vi "Configure AI Task.vi"(7 "Sampling Rate":dbl, 8 "error in (no error)":errorcluster, 11 "DAQ Tasks in":T1) -> (0 "error out":errorcluster, 3 "DAQ Tasks out":T1)   [LabVIEW 2015, in "DAQmx Module Runtime.lvclass"]
doc: "Configure AI Task by setting buffer to overwrite unread samples, setting sample clock, and starting the task."
uses:
  DAQmx Module Runtime.lvclass
  DAQ Tasks.ctl
  <vilib>/DAQmx/configure/timing.llb/DAQmx Timing (Sample Clock).vi
  <resource>/objmgr/daqmx.rc
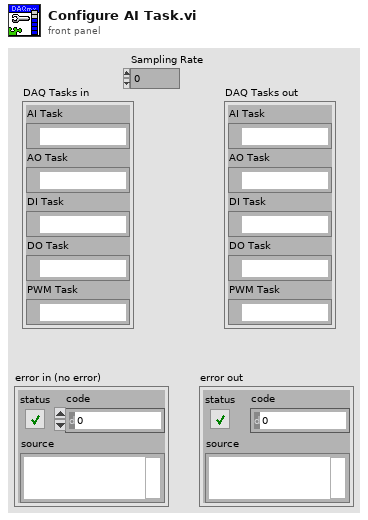
[diagram p1: front panel]
types:
  T1 = typedef "DAQmx Module Runtime.lvclass/DAQ Tasks.ctl" = cluster{"AI Task":refnum<k21>, "AO Task":refnum<k21>, "DI Task":refnum<k21>, "DO Task":refnum<k21>, "PWM Task":refnum<k21>}
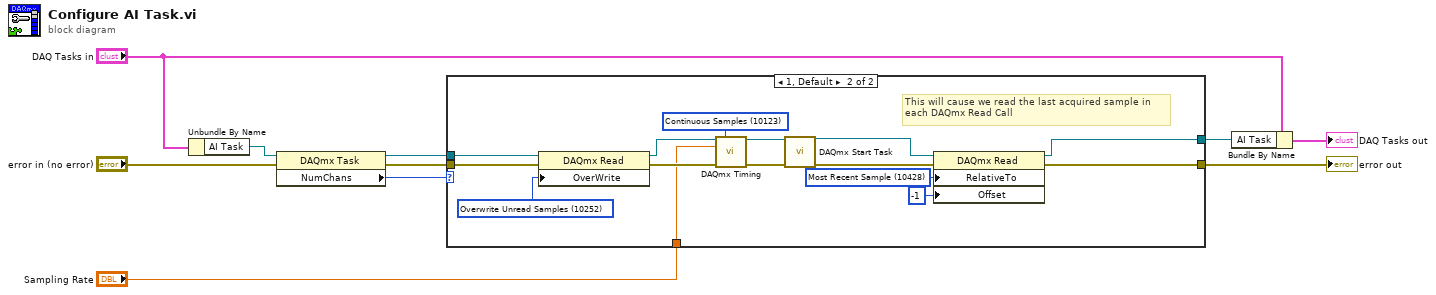
[diagram p0: block diagram]
diagram:
  n1 = Unbundle By Name("DAQ Tasks in") -> ("AI Task"=w2:refnum<k21>)
  n2 = property class="DAQmx Task"(reference=w2, error in="error in (no error)") -> (reference out=w9:refnum<k21>, error out=w7:errorcluster, "NumChans"=w6:u32)
  n3 = case shown="1, Default" w6 {
    tunnel: [w12 w14] -> w10
    tunnel: w9 -> [w11 w27]
    tunnel: w7 -> [w12 w26]
    tunnel: [w11 w13] -> w5
    tunnel: "Sampling Rate" -> [_ w19]
    frame 0 {
    }
    frame 1, Default {
      w18 = 10428 items=["First Sample"=10424, "Current Read Position"=10425, "Reference Trigger"=10426, "First Pretrigger Sample"=10427, "Most Recent Sample"=10428] ("RelativeTo")
      w20 = 10252 items=["Overwrite Unread Samples"=10252, "Do Not Overwrite Unread Samples"=10159] ("OverWrite")
      w25 = 10123 items=["Finite Samples"=10178, "Continuous Samples"=10123, "Hardware Timed Single Point"=12522] ("sample mode")
      # "This will cause we read the last acquired sample in\neach DAQmx Read Call"
      n4 = property class="DAQmx Read"(reference=w27, error in=w26, "OverWrite"=w20) -> (reference out=w21:refnum<k21>, error out=w22:errorcluster)
      n5 = call-poly <vilib>:"DAQmx Timing.vi"("task/channels in"=w21, "sample mode"=w25, "rate"=w19, "error in"=w22) -> ("task out"=w24:refnum<k21>, "error out"=w23:errorcluster)  [unwired: 10 in]
      n6 = call <vilib>:"DAQmx Start Task.vi"("task/channels in"=w24, "error in"=w23) -> ("task out"=w16:refnum<k21>, "error out"=w15:errorcluster)  [unwired: 12 in]
      n7 = property class="DAQmx Read"(reference=w16, error in=w15, "RelativeTo"=w18, "Offset"=-1) -> (reference out=w13:refnum<k21>, error out=w14:errorcluster)
    }
  }
  "error out" <- w10
  n8 = Bundle By Name(cluster="DAQ Tasks in", "AI Task"=w5) -> (→"DAQ Tasks out":T1)
